vi "Edge Detect.vi"(0 "Image Path":path=path "/Users/milandahal/Desktop/a.png", 5 "did":string="aa5f5cb08903b53f224287e0", 7 "wid":string="e1f73355bdbd9a727fdd999e", 9 "eid":string, 11 "Scaling Factor":dbl) -> (4 "Device Out":T2, 6 "Comm":T1, 8 "image":picture, 15 "error out":errorcluster)   [LabVIEW 2019]
uses:
  <userlib>/Onshape/_SubVI/Cluster.ctl
  <userlib>/IoT Devices/_subVIs/HTTPComm.ctl
  <userlib>/Onshape/_SubVI/z did wid and eid.vi
  <userlib>/ImageProcessing/InitCamera_NTSC.vi
  <userlib>/OnshapeFeatureFunctions/Onshape Feature Funcrions/_SubVI/FS Sketch Polyline.vi
panel:
  out "image 3":picture
  out "image 2":picture
  in  "stop":bool
  in  "Camera/ True or File/ False":bool=TRUE
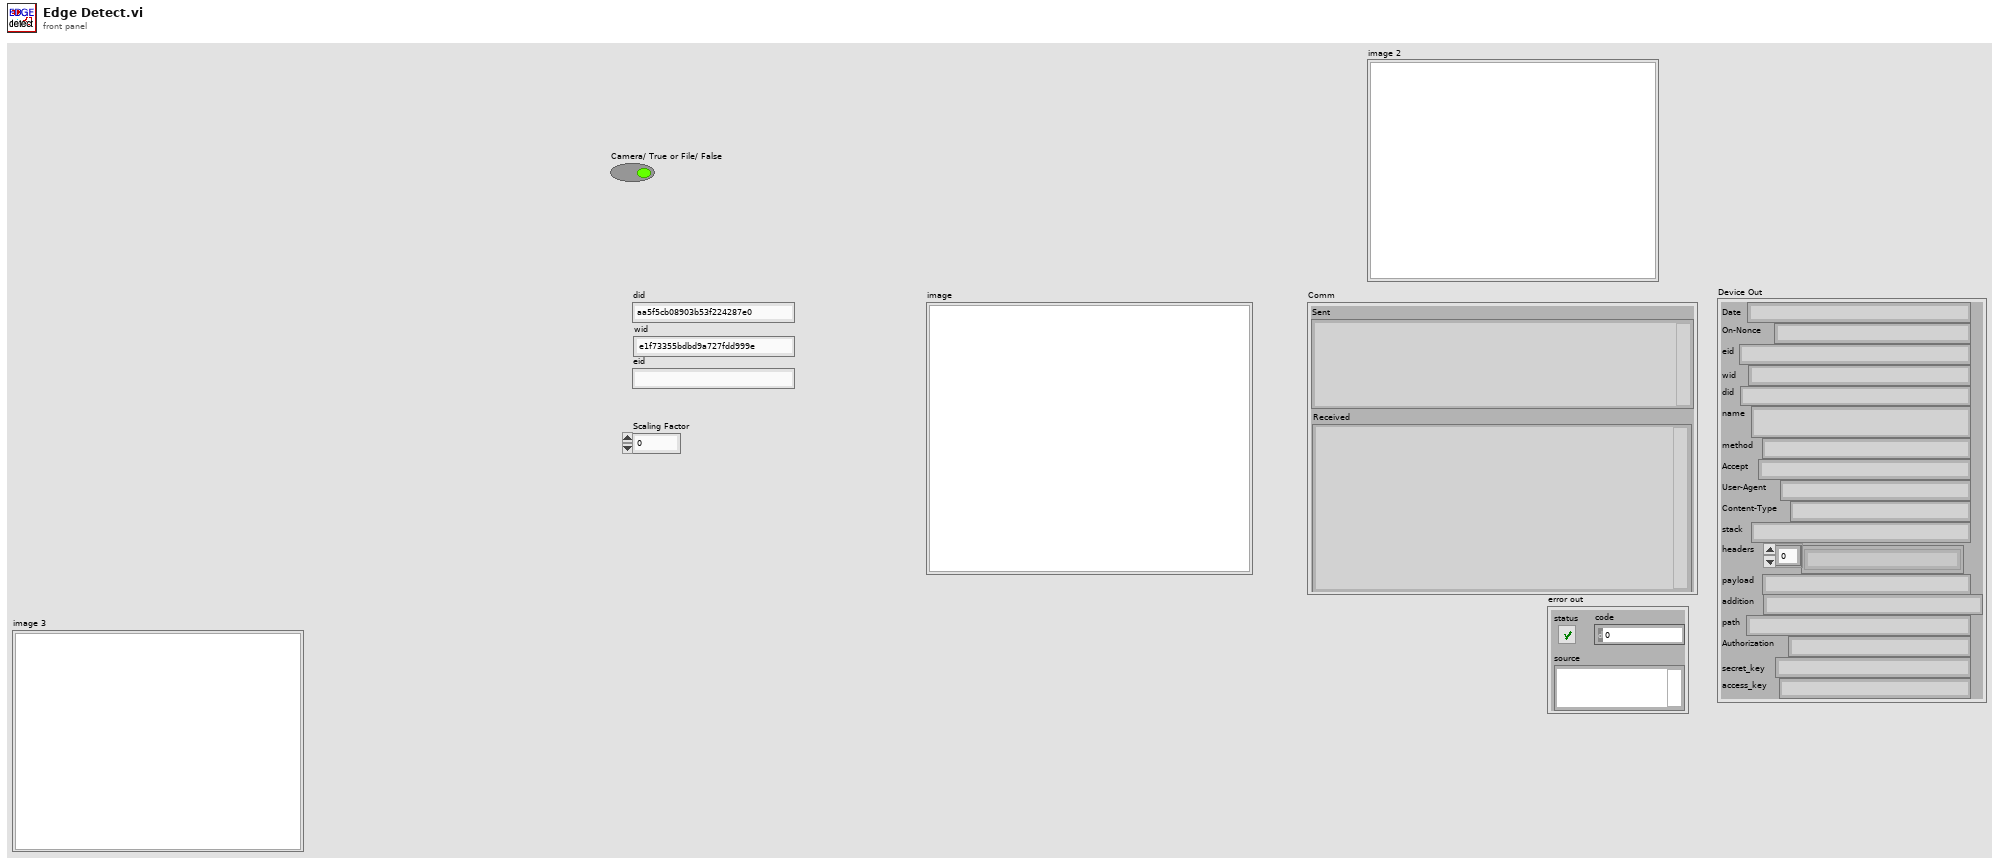
[diagram p1: front panel]
types:
  T1 = typedef "HTTPComm.ctl" = cluster{"url":string, "sent headers":string, "sent body":string, "headers":string, "body":string, "Sent":string, "Received":string}
  T2 = typedef "Cluster.ctl" = cluster{"Date":string, "On-Nonce":string, "eid":string, "wid":string, "did":string, "name":string, "method":string, "Accept":string, "User-Agent":string, "Content-Type":string, "stack":string, "headers":string[], "payload":string, "addition":string, "path":string, "Authorization":string, "secret_key":string, "access_key":string}
  T3 = typedef "QT_Image.ctl" = cluster{"Width":i32, "Height":i32, "Depth":i32, "data":u8[], "Compressed data":u8[], "Color table":u32[], "Duration":i32, "Options":i32, "Timestamp":i32, "ID":i32, "Reserved":i32, "Dialogs":u32}
  T4 = typedef "QT_Ref.ctl" = refnum<k1>
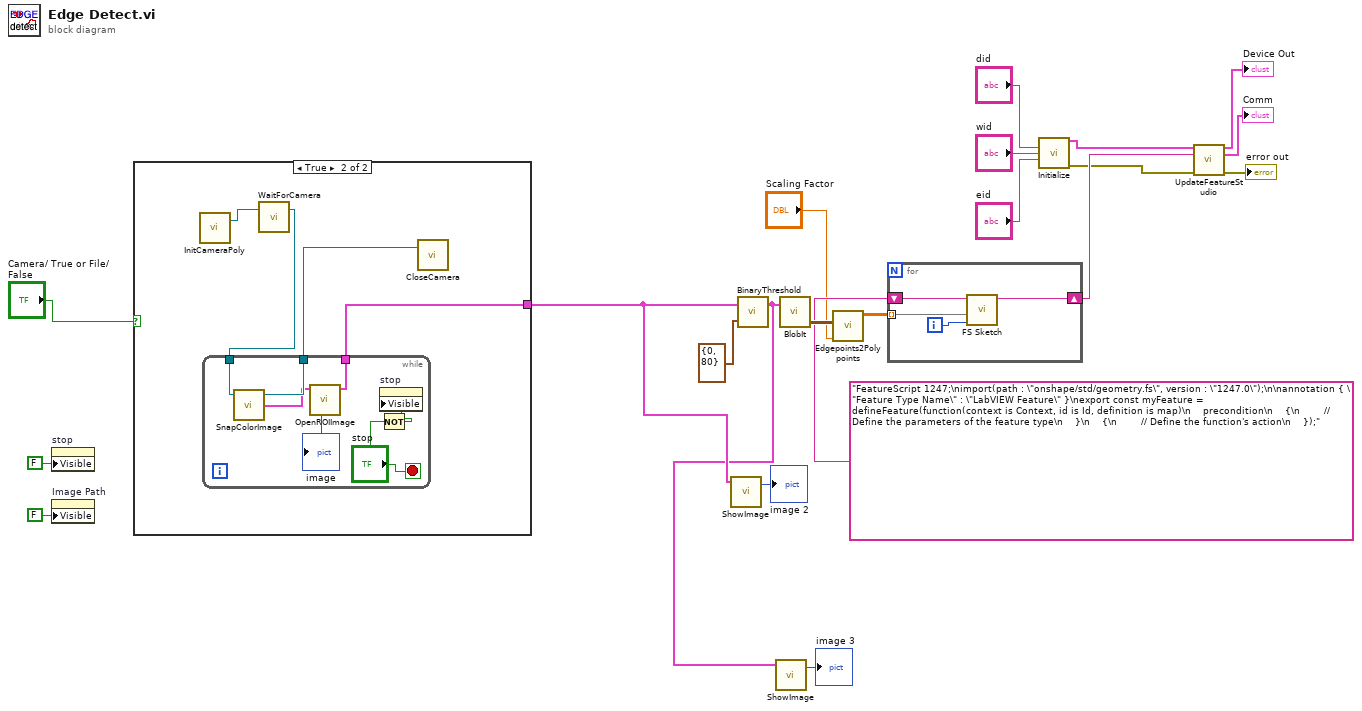
[diagram p0: block diagram]
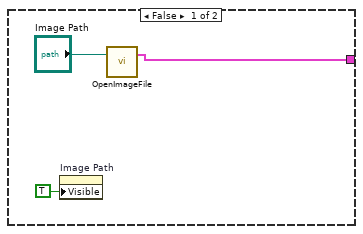
[diagram p2: hidden frame]
diagram:
  n1 = property on="stop" class="Bool"("Visible"=FALSE) -> ()  [unwired: 2 in, 2 out]
  n2 = property on="Image Path" class="Path"("Visible"=FALSE) -> ()  [unwired: 2 in, 2 out]
  n3 = case shown="True" "Camera/ True or File/ False" {
    tunnel: [w23 w25] -> w3
    frame False {
      n4 = property on="Image Path" class="Path"("Visible"=TRUE) -> ()  [unwired: 2 in, 2 out]
      n5 = call <userlib>:"OpenImageFile.vi"("selected path"="Image Path") -> ("Image Out"=w23:T3)  [unwired: 2 in]
    }
    frame True {
      n6 = call-poly <userlib>:"InitCameraPoly.vi"() -> ("QT Ref Out"=w28:T4)  [unwired: 2 in, 1 out]
      n7 = call <userlib>:"WaitForCamera.vi"("QT Ref In"=w28) -> ("QT Ref Out"=w27:T4)  [unwired: 1 in, 1 out]
      n8 = while {
        tunnel: w27 -> [w33]
        tunnel: [w32] -> w26
        tunnel: [w30] -> w25
        stop <- "stop" stop-if-true
        n9 = call <userlib>:"SnapColorImage.vi"("QT Ref In"=w33) -> ("Image Out"=w31:T3, "QT Ref Out"=w32:T4)  [unwired: 2 in, 1 out]
        n10 = call "OpenROIImage.vi"("Image  in"=w31) -> ("image"=→"image":picture, "Image  out"=w30:T3)  [unwired: 9 in]
        n11 = Not(x="stop") -> (.not. x?=w34:bool)
        n12 = property on="stop" class="Bool"("Visible"=w34) -> ()  [unwired: 2 in, 2 out]
      }
      n13 = call <userlib>:"CloseCamera.vi"("QT Ref In"=w26) -> ()  [unwired: 2 in, 1 out]
    }
  }
  n14 = call <userlib>:"ShowImage.vi"("Image"=w3) -> ("image"=→"image 2":picture)  [unwired: 2 in, 1 out]
  n15 = call <userlib>:"BinaryThreshold.vi"("threshold"=cluster{u8, u8} {0, 80}, "Image In"=w3) -> ("Image Out"=w1:T3)  [unwired: 1 in]
  n16 = call <userlib>:"ShowImage.vi"("Image"=w1) -> ("image"=→"image 3":picture)  [unwired: 2 in, 1 out]
  n17 = call <userlib>:"BlobIt.vi"("Image in"=w1) -> ("Array 2"=w21:cluster{"Row":i32, "Col":i32}[][])  [unwired: 1 in, 2 out]
  n18 = call <userlib>:"Edgepoints2Polypoints.vi"("Scaling Factor"="Scaling Factor", "Edgepoints In"=w21) -> ("Polyline Out"=w20:dbl[][][])  [unwired: 9 in]
  n19 = for {
    tunnel: w20 -> [w39] mode=indexing
    shift-right: [w36] -> w15
    shift-left: "FeatureScript 1247;\nimport(path : \"onshape/std/geometry.fs\", version : \"1247.0\");\n\nannotation { \"Feature Type Name\" : \"LabVIEW Feature\" }\nexport const myFeature = defineFeature(function(context is Context, id is Id, definition is map)\n    precondition\n    {\n        // Define the parameters of the feature type\n    }\n    {\n        // Define the function's action\n    });" ("Feature In") -> [w37]
    i -> [w38]
    n20 = call-poly <userlib>:"FS Sketch.vi"("Sketch #"=w38, "Polyline Points"=w39, "Feature In"=w37) -> ("Feature Out"=w36:string)  [unwired: 8 in]
  }
  n21 = call-poly <userlib>:"Initialize.vi"("did"="did", "wid"="wid", "eid"="eid") -> ("Device Out"=w16:T2, "error out"=w8:errorcluster)  [unwired: 11 in]
  n22 = call <userlib>:"UpdateFeatureStudio.vi"("Device In"=w16, "FeatureScript"=w15, "error in"=w8) -> ("Device Out"=→"Device Out":T2, "Comm"=→"Comm":T1, "error out"=→"error out":errorcluster)  [unwired: 10 in]
